vi "Timed Loop Resettable Source Type.vi"() -> ()   [LabVIEW 2023]
doc: "This VI illustrates the difference between timed loops with non-resettable timing sources and timed loops with resettable timing sources. Simply select the number of loop resets you wish to simulate along with the number of loop iterations to execute before each reset, and the timing results will be plotted on the front panel graphs."
uses:
  <vilib>/Platform/TimedLoop/XDataNode/timing_clust.ctl
  <vilib>/Platform/TimedLoop/XDataNode/nitl_modes.ctl
  <vilib>/Platform/TimedLoop/XDataNode/wakeup.ctl
  <vilib>/platform/TimedLoop/XDataNode/XDataNode.xnode
  <vilib>/Platform/TimedLoop/XDataNode/XDNodeRunTimeDep.lvlib
panel:
  out "Start Times (non-resettable)":i64[](graph)
  out "Start Times (resettable)":i64[](graph)
  # "Overview: Demonstrates a resettable Source Type timing source configuration on a Timed Loop.\nRequirements: Windows\nInstructions:\nRun the VI. Observe the different Iteration Start Times between the two loop configurations. See the block diagram for more information."
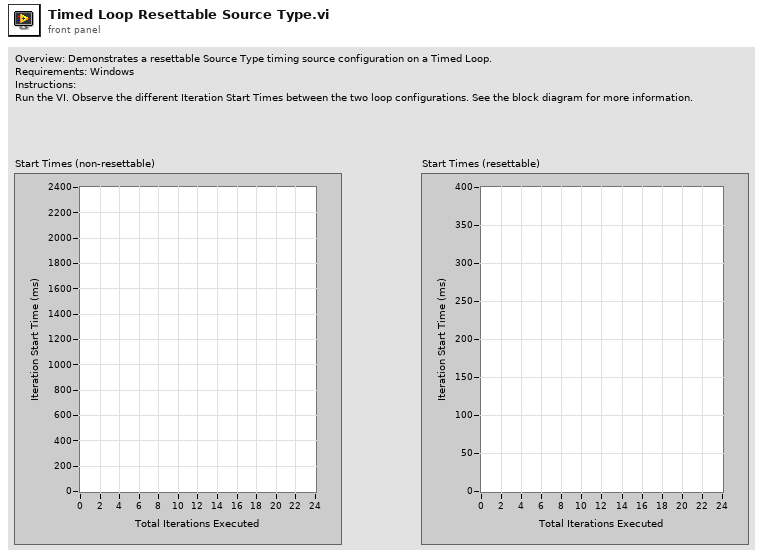
[diagram p1: front panel]
types:
  T1 = typedef "XDNodeRunTimeDep.lvlib/timing_clust.ctl" = cluster{"Expected End [f-1]":u64, "Actual End [f-1]":u64, "Finished Late? [f-1]":bool, "Expected End [i-1]":u64, "Actual End [i-1]":u64, "Finished Late? [i-1]":bool, "Expected Start [i]":u64, "Actual Start [i]":u64, "Expected Start [f]":u64, "Actual Start [f]":u64, "Source Name":string, "Structure Name":string, "Period":i64, "Deadline":i64, "Offset":i64, "Start":i64, "Priority":i32, "Timeout":i32, "Mode":T2, "Wakeup Reason":T3, "Error":errorcluster, "Source Type":string, "Secondary Source Type":string, "Global End Time":u64, "Global Start Time":u64, "Frame Duration":u64, "Iteration Duration":u64, "Assigned CPU":i32, "I/O Scan Engine Mode":u32}
  T2 = typedef "XDNodeRunTimeDep.lvlib/nitl_modes.ctl" = enum32{"No Change", "Process missed periods, maintain original phase", "Discard missed periods, maintain original phase", "Process missed periods, ignore original phase", "Discard missed periods, ignore original phase"}
  T3 = typedef "XDNodeRunTimeDep.lvlib/wakeup.ctl" = enum32{"Normal", "Aborted", "Asynchronous wakeup", "Timing source error", "Timed loop error", "Timeout"}
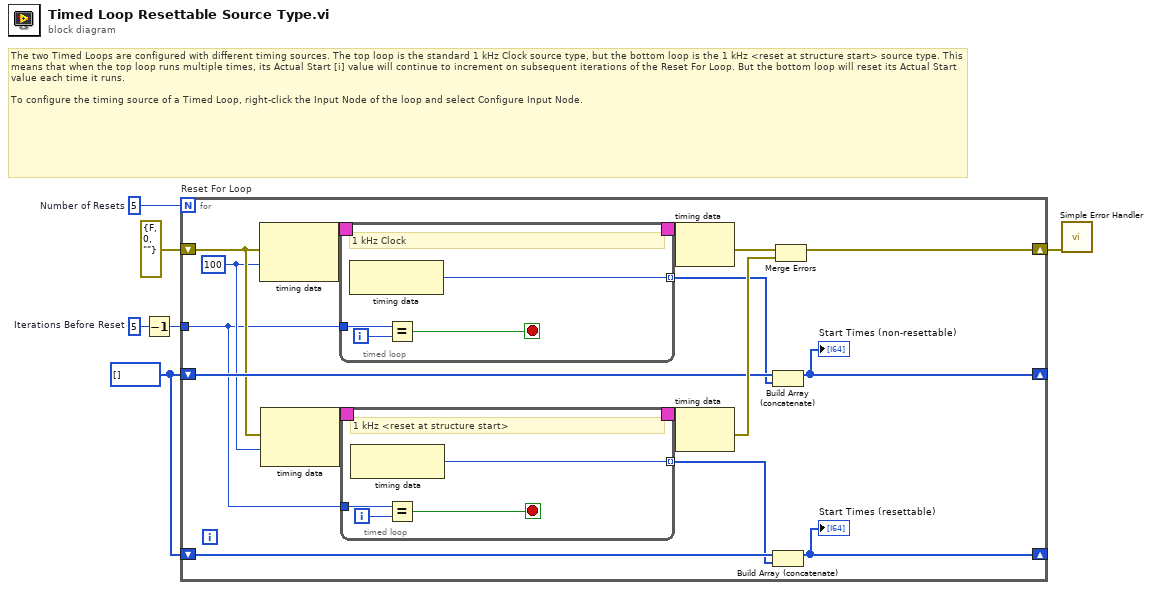
[diagram p0: block diagram]
diagram:
  w2 = 5  # Iterations Before Reset
  w4 = 5  # Number of Resets
  w5 = i64[] []
  # "The two Timed Loops are configured with different timing sources. The top loop is the standard 1 kHz Clock source type, but the bottom loop is the 1 kHz <reset at structure start> source type. This means that when the top loop runs multiple times, its Actual Start [i] value will continue to increment on subsequent iterations of the Reset For Loop. But the bottom loop will reset its Actual Start value each time it runs.\n\nTo configure the timing source of a Timed Loop, right-click the Input Node of the loop and select Configure Input Node."
  n1 = Decrement(x=w2) -> (x-1=w1:i32)
  n2 = for "Reset For Loop" {
    N: w4 -> [_]
    shift-right: [w16] -> w6
    shift-left: errorcluster {"status"=FALSE, "code"=0, "source"=""} ("error constant") -> [w9]
    shift-right: [w14] -> _
    shift-left: w5 -> [w15]
    shift-right: [w10] -> _
    shift-left: w5 -> [w12]
    tunnel: w1 -> [w7]
    w8 = i64 100 ("Period")
    n3 = node-c288(w9, w8) -> (w20:T1)
    n4 = node-c288(w9, w8) -> (w22:T1)
    n5 = timed-loop "Non-Resettable" {
      timing: w20 -> [_]
      timing-out: [_] -> w19
      tunnel: w7 -> [w25]
      tunnel: [w24] -> w13 mode=indexing
      i -> [w26]
      stop <- w23 stop-if-true
      # "1 kHz Clock"
      n6 = node-c288() -> (w24:i64)  [unwired: 1 in]
      n7 = Equal?(x=w25, y=w26) -> (x = y?=w23:bool)
    }
    n8 = timed-loop "Resettable" {
      timing: w22 -> [_]
      timing-out: [_] -> w21
      tunnel: w7 -> [w38]
      tunnel: [w37] -> w11 mode=indexing
      i -> [w39]
      stop <- w36 stop-if-true
      # "1 kHz <reset at structure start>"
      n9 = node-c288() -> (w37:i64)  [unwired: 1 in]
      n10 = Equal?(x=w38, y=w39) -> (x = y?=w36:bool)
    }
    n11 = node-c288(w19) -> (w18:errorcluster)
    n12 = node-c288(w21) -> (w17:errorcluster)
    n13 = Build Array (concatenate)(w15, w13) -> (w14:i64[])
    "Start Times (non-resettable)" <- w14
    n14 = Build Array (concatenate)(w12, w11) -> (w10:i64[])
    "Start Times (resettable)" <- w10
    n15 = Merge Errors(w18, w17) -> (w16:errorcluster)
  }
  n16 = call <vilib>:"Simple Error Handler.vi"("error in (no error)"=w6) -> ()  [unwired: 4 in, 5 out]
